vi "Get ProtoFile Oneofs.vi"(8 "error in (no error)":errorcluster, 10 "ProtoFile Messages":u64[](array[numeric]), 11 "Protofile ref in":u64) -> (0 "error out":errorcluster, 2 "ProtoFile Oneofs":u64[](array[numeric]), 3 "Protofile ref out":u64)   [LabVIEW 2019, in "gRPC Template Creation Utility.lvlib"]
uses:
  gRPC Template Creation Utility.lvlib
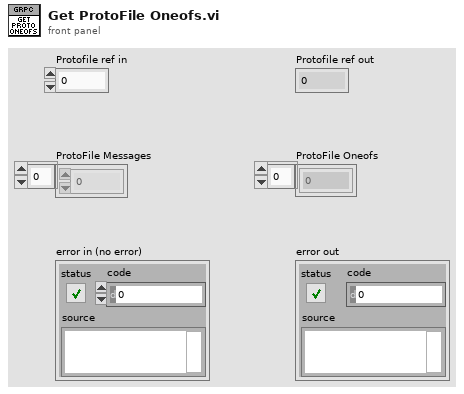
[diagram p1: front panel]
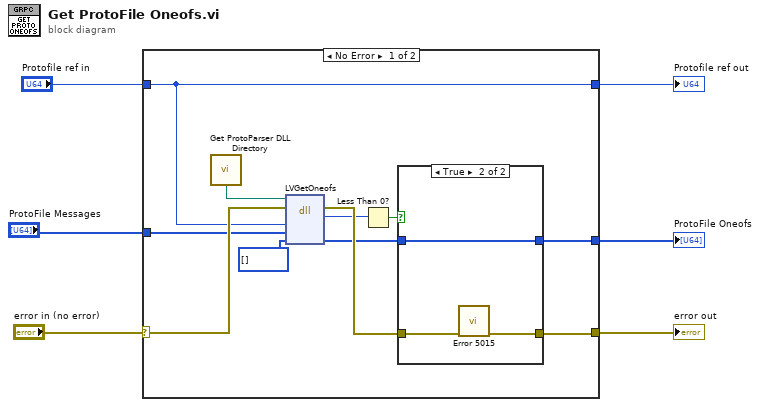
[diagram p0: block diagram]
diagram:
  n1 = case shown="No Error" "error in (no error)" {
    selector: "error in (no error)" -> [w16 w23]
    tunnel: "Protofile ref in" -> [w15 w24]
    tunnel: [w15 w24] -> w4
    tunnel: [w14 w23] -> w3
    tunnel: [w10 _] -> w2
    tunnel: "ProtoFile Messages" -> [w7 _]
    frame No Error {
      n2 = call "Get ProtoParser DLL Directory.vi"() -> ("Proto Parser Directory"=w17:path)
      n3 = dll-call lib="C:/Source/grpc-labview/build/Debug/labview_grpc_generator.dll" fn="LVGetOneofs"(path in=w17, error in=w16, "protoDescription"=w15, "messages"=w7, "oneofs"=u64[] []) -> (error out=w13:errorcluster, "return type"=w12:i32, "oneofs"=w8:u64[])  [unwired: 3 in, 1 out]
      n4 = Less Than 0?(x=w12) -> (x < 0?=w11:bool)
      n5 = case shown="True" w11 {
        tunnel: [w18 w22] -> w14
        tunnel: w13 -> [w18 w21]
        tunnel: w8 -> [w19 w20]
        tunnel: [w19 w20] -> w10
        frame False {
        }
        frame True {
          n6 = call "Error 5015.vi"("error in (no error)"=w21) -> ("error out"=w22:errorcluster)  [unwired: 10 in]
        }
      }
    }
    frame Error {
    }
  }
  "ProtoFile Oneofs" <- w2
  "Protofile ref out" <- w4
  "error out" <- w3
